vi "Set_Still_Power.vi"(8 "VISA session":refnum<visa-resource-name>="GPIB0::17::INSTR", 9 "Still Heater Resistance (mW)":dbl, 10 "Still Power (mW)":dbl, 11 "Still heater":bool) -> ()   [LabVIEW 2016]
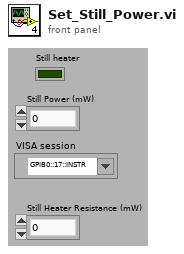
[diagram p1: front panel]
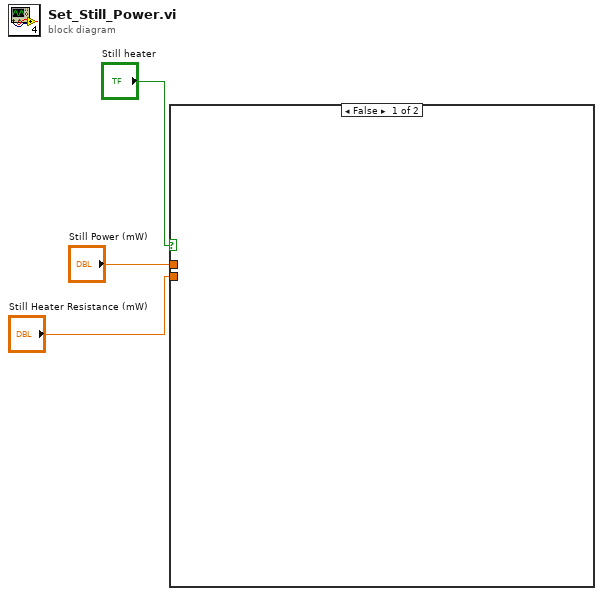
[diagram p0: block diagram]
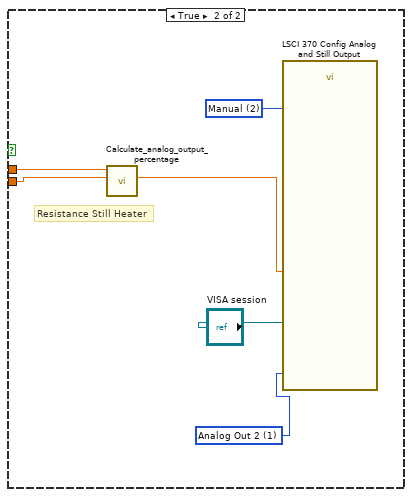
[diagram p2: hidden frame]
diagram:
  n1 = case shown="False" "Still heater" {
    tunnel: "Still Power (mW)" -> [_ w9]
    tunnel: "Still Heater Resistance (mW)" -> [_ w8]
    frame False {
    }
    frame True {
      w6 = u16 1 items=["Analog Out 1", "Analog Out 2"] ("Analog Channel (0: Analog Out 1)")
      w5 = u16 2 items=["Off", "Channel", "Manual", "Zone", "Still"] ("Analog Out Mode (0: Off)")
      # "Resistance Still Heater"
      n2 = call "Calculate_analog_output_percentage.vi"("Resistance (Ohms)"=w8, "Power (mW)"=w9) -> ("Analog Output (%)"=w4:dbl)  [unwired: 9 in]
      n3 = call "LSCI 370 Config Analog and Still Output.vi"("VISA session"="VISA session", "Analog Out Mode (0: Off)"=w5, "Analog Channel (0: Analog Out 1)"=w6, "Manual Value (0.000)"=w4) -> ()  [unwired: 10 in, 2 out]
    }
  }
